vi "WRITE CAN.vi"() -> ()   [LabVIEW 2018]
uses:
  <vilib>/xnet/xnet.llb/XNET Create Session (Frame Input Stream).vi
  <vilib>/xnet/xnet.llb/XNET Read (Frame CAN).vi
  <resource>/objmgr/xnet.rc
panel:
  in  "stop":bool
  out "Frames":string[][](table)
  in  "Hex Display":bool
  in  "Number of Frames to Display":i32=15
  in  "CAN Cluster":refnum<k21>=":memory:"
  in  "BaudRate":u32=125000
  in  "Select Interface":refnum<k21>="CAN2"
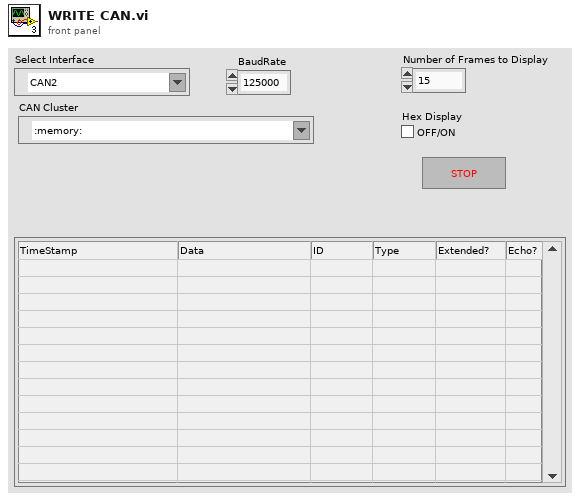
[diagram p1: front panel]
types:
  T1 = typedef "XNET Frame CAN.ctl" = cluster{"timestamp":timestamp, "payload":u8[], "identifier":u32, "type":T2, "extended?":bool, "echo?":bool}
  T2 = typedef "XNET Frame Type CAN.ctl" = u8
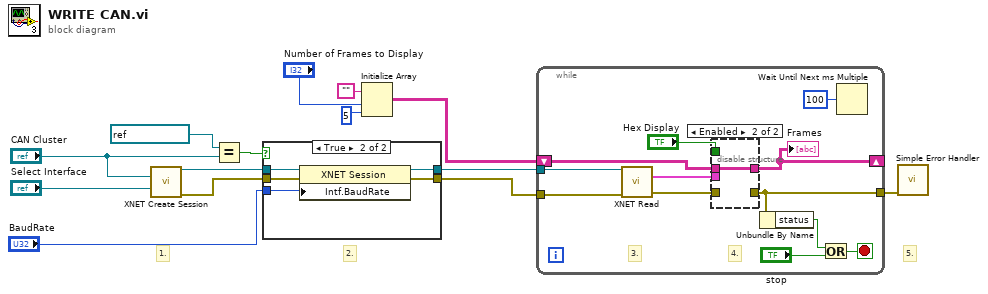
[diagram p0: block diagram]
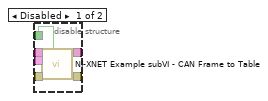
[diagram p2: hidden frame]
diagram:
  # "2."
  # "5."
  # "1."
  n1 = call-poly <vilib>:"XNET Create Session.vi"("cluster (:memory:)"="CAN Cluster", "interface"="Select Interface") -> ("session out"=w12:refnum<k21>, "error out"=w8:errorcluster)  [unwired: 1 in, 11 out]
  n2 = Equal?(x=refnum<k21> ":memory:" ("CAN Cluster"), y="CAN Cluster") -> (x = y?=w7:bool)
  n3 = case shown="True" w7 {
    tunnel: w12 -> [w16 w21]
    tunnel: [w16 w20] -> w11
    tunnel: "BaudRate" -> [_ w19]
    tunnel: [w15 w18] -> w9
    tunnel: w8 -> [w15 w17]
    frame False {
    }
    frame True {
      n4 = property class="XNET Session"(reference=w21, error in=w17, "Intf.BaudRate"=w19) -> (reference out=w20:refnum<k21>, error out=w18:errorcluster)
    }
  }
  n5 = Initialize Array("", "Number of Frames to Display", 5 ("Dimension Size")) -> (w1:string[][])
  n6 = while {
    tunnel: w11 -> [w33]
    tunnel: w9 -> [w32]
    tunnel: [w24] -> w13
    shift-right: [w26] -> _
    shift-left: w1 -> [w28]
    stop <- w29 stop-if-true
    # "4."
    # "3."
    n7 = call-poly <vilib>:"XNET Read.vi"("session in"=w33, "error in (no error)"=w32) -> ("data"=w27:T1[], "error out"=w25:errorcluster)  [unwired: 12 out]
    n8 = disable-structure shown="Enabled" {
      disable-tunnel: w28 -> [w39 w40]
      disable-tunnel: w27 -> [w38 _]
      disable-tunnel: [w37 w40] -> w26
      disable-tunnel: w25 -> [w36 _]
      disable-tunnel: [w35 _] -> w24
      disable-tunnel: "Hex Display" -> [w34 _]
      frame Disabled {
        n9 = call "NI-XNET Example subVI - CAN Frame to Table.vi"("Hexadecimal?"=w34, "error in (no error)"=w36, "CAN Frames (from XNET Read)"=w38, "Input Array"=w39) -> ("error out"=w35:errorcluster, "Output Array"=w37:string[][])  [unwired: 1 in, 5 out]
      }
      frame Enabled {
      }
    }
    "Frames" <- w26
    n10 = Unbundle By Name(w24) -> ("status"=w31:bool)
    n11 = Or(x=w31, y="stop") -> (x .or. y?=w29:bool)
    n12 = Wait Until Next ms Multiple(millisecond multiple=u32 100 ("milliseconds to wait")) -> ()  [unwired: 1 out]
  }
  n13 = call <vilib>:"Simple Error Handler.vi"("error in (no error)"=w13) -> ()  [unwired: 1 in, 8 out]
